vi "ATF Drive and PPSU Feedback.vi"() -> ()   [LabVIEW 2022 SP3]
uses:
  <vilib>/Analysis/baseanly.llb/Mean (DBL).vi
  <vilib>/Analysis/NI_AALBase.lvlib
panel:
  in  "Exit":bool
  out "Deceleration State":bool
  out "Steady State":bool
  out "Accereleration State":bool
  out "C-Phase short circuit":bool
  out "B-Phase short circuit":bool
  out "Motor Winding\n Short circuit or Overload":bool
  out "Speed command &\n response mismatch":bool
  out "C-Phase bottom \nMOSFETshort circuit":bool
  out "C-Phase top\n MOSFET short circuit":bool
  out "B-Phase bottom \nMOSFET short circuit":bool
  out "B-Phase top\n MOSFET short circuit":bool
  out "A-Phase bottom\n MOSFET short  circuit":bool
  out "A-Phase top \nMOSFET short circuit":bool
  out "Over speed":bool
  out "A-Phase short circuit":bool
  out "C-Phase open circuit":bool
  out "B-Phase open circuit":bool
  out "A-Phase open circuit":bool
  out "C-Phase bottom\n MOSFET open circuit":bool
  out "C-Phase top\n MOSFET open circuit":bool
  out "B-Phase bottom \nMOSFET open circuit":bool
  out "B-Phase top \nMOSFET open circuit":bool
  out "A-Phase bottom \nMOSFETopen circuit":bool
  out "A-Phase top\n MOSFET open circuit":bool
  out "Over Temperature":bool
  out "Drive Health":bool
  out "Shaft Rotational Direction":string
  out "Running Frequency":dbl format="%.2f"
  out "Run_Acknowledgement":bool
  out "Speed (RPM)":dbl format="%.2f"
  out "DC Busbar":dbl format="%.2f"
  out "DC Busbar":dbl format="%.2f"
  out "DC Busbar":dbl format="%.2f"
  out "Leg3 Cooling Jacket":dbl format="%.2f"
  out "Leg3 Cooling Jacket":dbl format="%.2f"
  out "Leg2 Cooling Jacket":dbl format="%.2f"
  out "Leg2 Cooling Jacket":dbl format="%.2f"
  out "Leg1 Cooling Jacket":dbl format="%.2f"
  out "Ic,ph,mean":dbl format="%.2f"
  out "Ib,ph,mean":dbl format="%.2f"
  out "Ia,ph,mean":dbl format="%.2f"
  out "Vc,ph,mean":dbl format="%#.2f"
  out "Vb,ph,mean":dbl format="%#.2f"
  out "Va,ph,mean":dbl format="%#.2f"
  out "Ic,ph,rms":dbl format="%.2f"
  out "Ib,ph,rms":dbl format="%.2f"
  out "Ia,ph,rms":dbl format="%.2f"
  out "Idc (A)":dbl format="%.2f"
  out "Vc,ph,rms":dbl format="%.2f"
  out "Vb,ph,rms":dbl format="%.2f"
  out "Va,ph,rms":dbl format="%.2f"
  out "Vdc (V)":dbl format="%.2f"
  # "ATF DRIVE AND PPSU FEEDBACK"
  # "DRIVE HEALTH & FEED BACK"
  # "FAULT STATUS"
  # "Drive Critical Parameters"
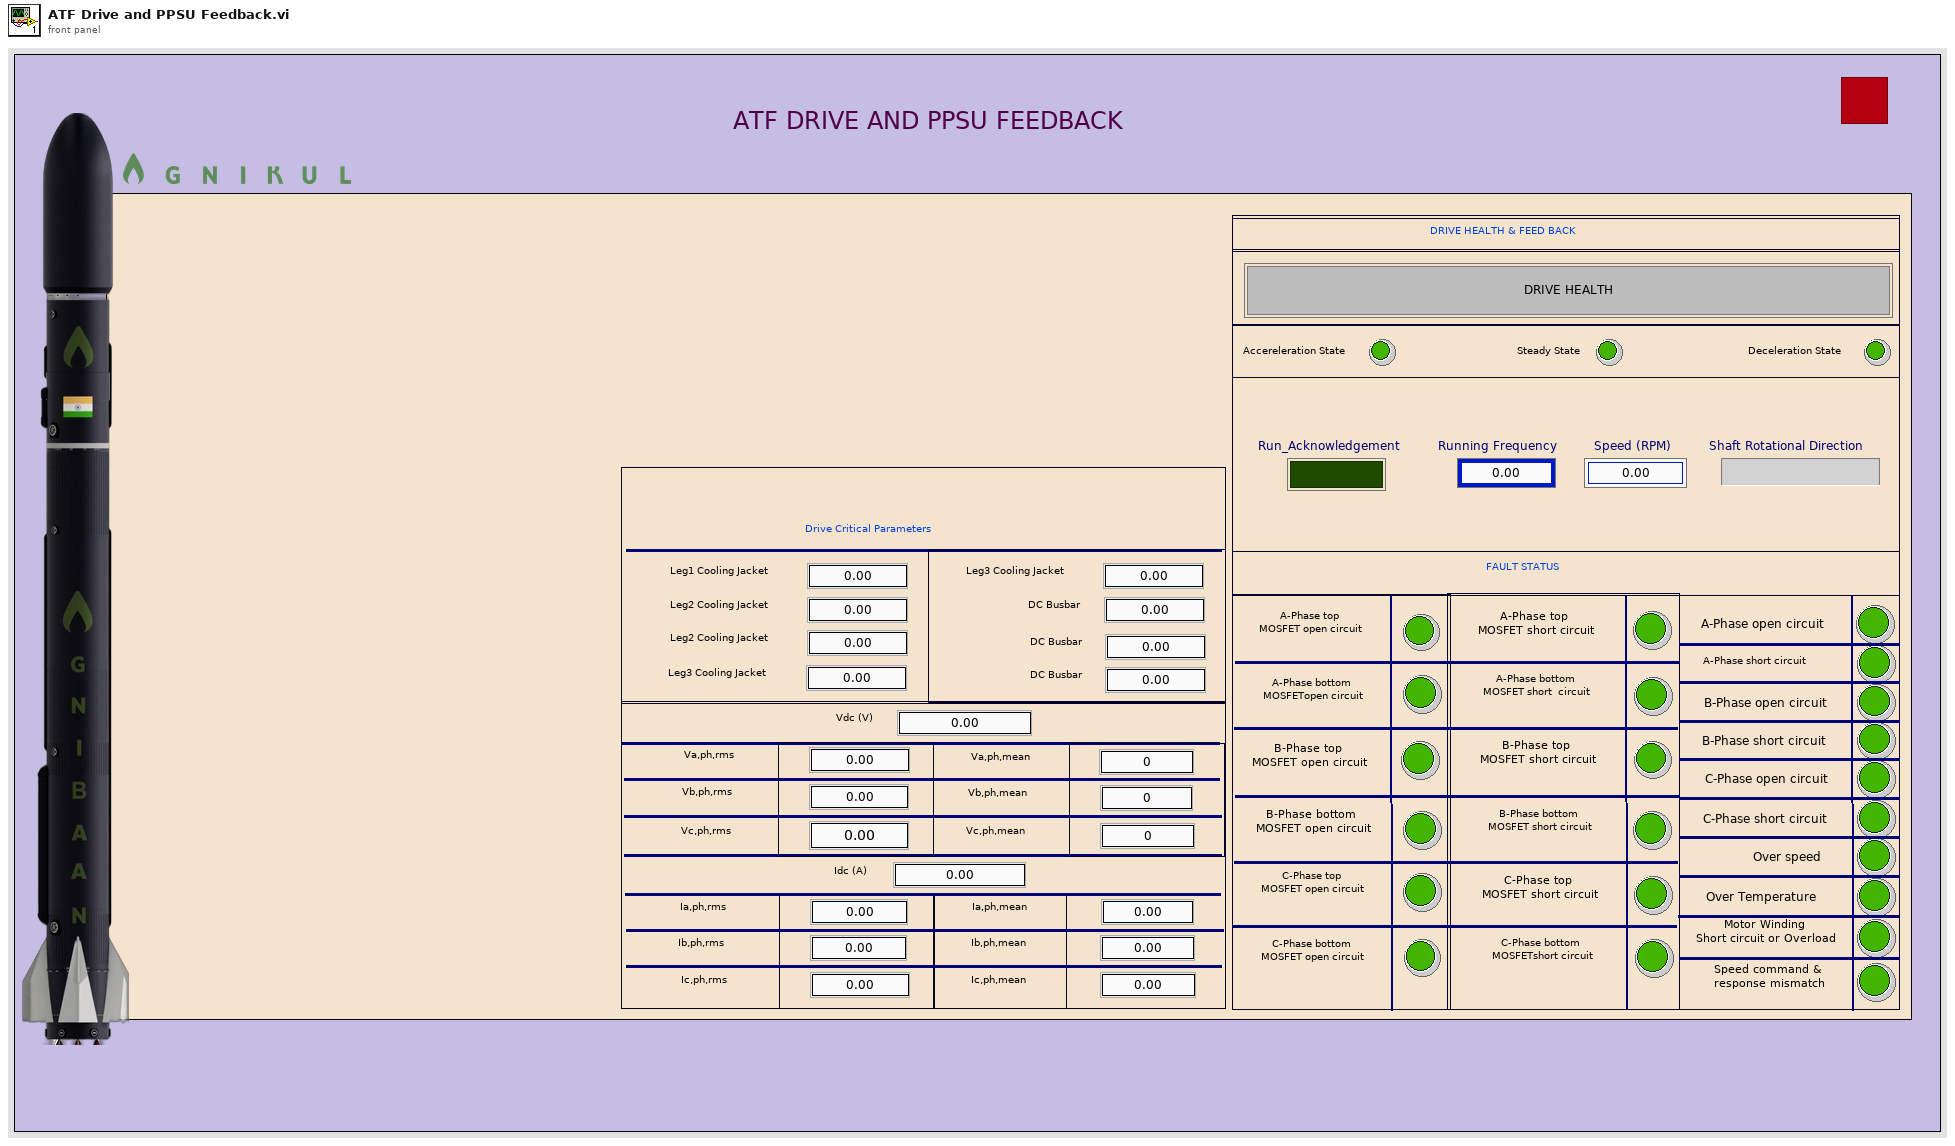
[diagram p1: front panel]
types:
  T1 = typedef "SeCrTS-Notifier Ref.ctl" = cluster{"Pump":refnum<notifier>, "Storage":refnum<notifier>}
  T2 = cluster{"AI_V_Data":waveform(dbl)[][], "AI_C_Data":waveform(dbl)[][], "AO_Data":waveform(dbl)[][], "DO_Data":waveform(dbl)[][], "DI_Data":digitalwaveform[][], "ACC_Data":waveform(dbl)[][], "TC Data":waveform(dbl)[][], "Drive_A_C":waveform(dbl)[][], "Drive_A_D":waveform(dbl)[][], "AI_V Rms":waveform(dbl)[][]}
  T3 = cluster{"Drive_Health":bool, "Drive_Frequency":u32, "Drive_Status":bool, "Drive_RPM":u32, "Drive_Direction":bool, "Acceleration state":bool, "Steady state":bool, "Deceleration state":bool, "Drive_Enable":bool, "Drive set_RPM":dbl}
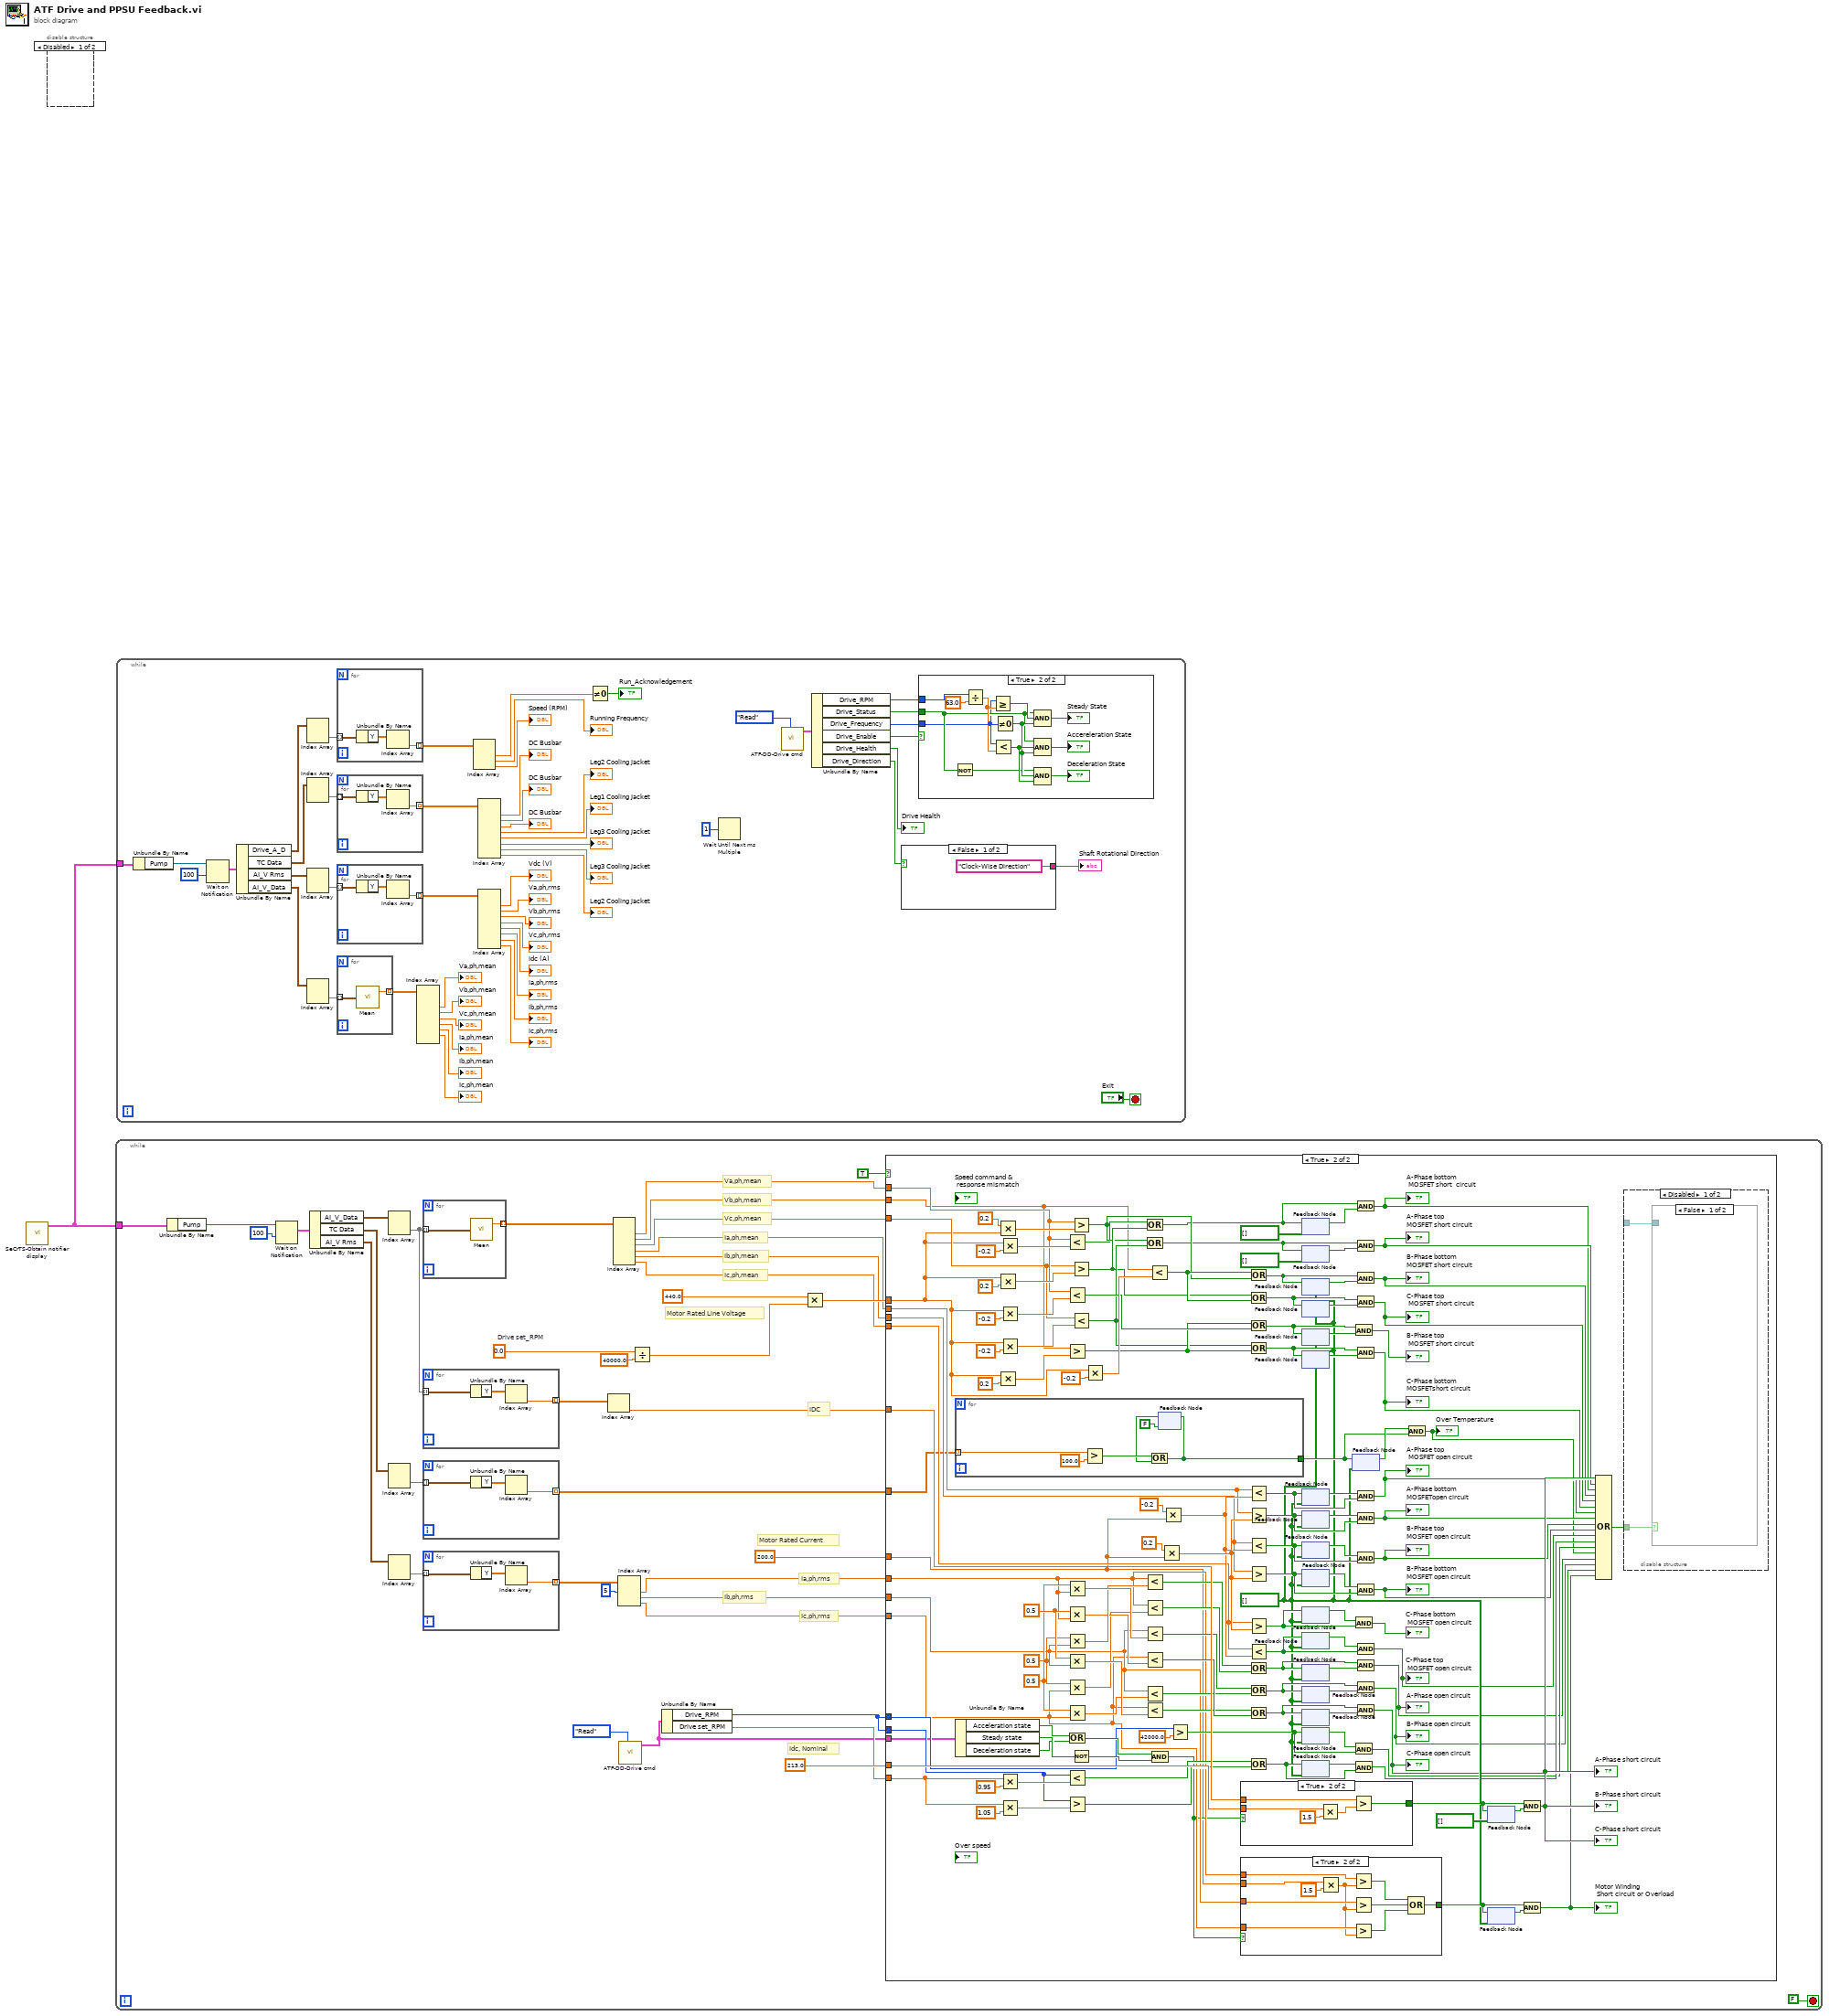
[diagram p0: block diagram]
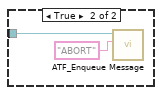
[diagram p3: hidden frame]
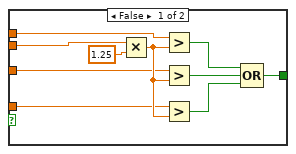
[diagram p5: hidden frame]
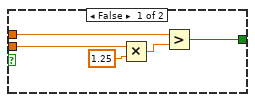
[diagram p6: hidden frame]
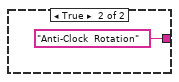
[diagram p9: hidden frame]
diagram:
  n1 = call "SeCrTS-Obtain notifier display.vi"() -> ("NOT DIS Out"=w1:T1)  [unwired: 10 in, 1 out]
  n2 = disable-structure shown="Disabled" {
    frame Disabled {
    }
    frame Enabled {
    }
  }
  n3 = while {
    tunnel: w1 -> [w31]
    stop <- FALSE ("UI Exit") stop-if-true
    w26 = 0.0  # Drive set_RPM
    # "Ic,ph,rms"
    # "Ib,ph,rms"
    # "Ia,ph,rms"
    # "Ic,ph,mean"
    # "Ib,ph,mean"
    # "Ia,ph,mean"
    # "Vb,ph,mean"
    # "Vc,ph,mean"
    # "Va,ph,mean"
    # "IDC"
    # "Idc, Nominal"
    # "Motor Rated Line Voltage"
    # "Motor Rated Current"
    n4 = Unbundle By Name(w31) -> ("Pump"=w30:refnum<notifier>)
    n5 = Wait on Notification(notifier=w30, timeout in ms (-1)=100) -> (notification=w29:T2)  [unwired: 2 in, 3 out]
    n6 = Unbundle By Name(w29) -> ("AI_V_Data"=w28:waveform(dbl)[][], "TC Data"=w25:waveform(dbl)[][], "AI_V Rms"=w13:waveform(dbl)[][])
    n7 = Index Array(array=w28) -> (element=w21:waveform(dbl)[])  [unwired: 2 in]
    n8 = Index Array(array=w25) -> (element=w24:waveform(dbl)[])  [unwired: 2 in]
    n9 = Index Array(array=w13) -> (element=w12:waveform(dbl)[])  [unwired: 2 in]
    n10 = for {
      tunnel: w21 -> [w44] mode=indexing
      tunnel: [w43] -> w20 mode=indexing
      n11 = call-poly <vilib>:"Mean.vi"("X"=w44) -> ("mean"=w43:dbl)  [unwired: 1 out]
    }
    n12 = for {
      tunnel: w21 -> [w47] mode=indexing
      tunnel: [w45] -> w22 mode=indexing
      n13 = Unbundle By Name(w47) -> ("Y"=w46:dbl[])
      n14 = Index Array(array=w46) -> (element=w45:dbl)  [unwired: 1 in]
    }
    n15 = for {
      tunnel: w24 -> [w50] mode=indexing
      tunnel: [w48] -> w35 mode=indexing
      n16 = Unbundle By Name(w50) -> ("Y"=w49:dbl[])
      n17 = Index Array(array=w49) -> (element=w48:dbl)  [unwired: 1 in]
    }
    n18 = for {
      tunnel: w12 -> [w42] mode=indexing
      tunnel: [w40] -> w11 mode=indexing
      n19 = Unbundle By Name(w42) -> ("Y"=w41:dbl[])
      n20 = Index Array(array=w41) -> (element=w40:dbl)  [unwired: 1 in]
    }
    n21 = Index Array(array=w22) -> (element=w27:dbl)  [unwired: 1 in]
    n22 = Index Array(array=w20) -> (element #1=w19:dbl, element #2=w18:dbl, element #3=w17:dbl, element #4=w16:dbl, element #5=w15:dbl, element #6=w14:dbl)  [unwired: 6 in]
    n23 = Index Array(array=w11, index #1=5 ("index")) -> (element #1=w9:dbl, element #2=w8:dbl, element #3=w7:dbl)  [unwired: 2 in]
    n24 = call "ATF-DD-Drive cmd.vi"("Enum"=enum16{"Read", "Write"}."Read") -> ("Data.Drive 2"=w2:T3)  [unwired: 9 in, 1 out]
    n25 = Divide(x=w26, y=40000.0) -> (x/y=w37:dbl)
    n26 = Unbundle By Name(w2) -> ("Drive_RPM"=w6:u32, "Drive set_RPM"=w5:dbl)
    n27 = Multiply(x=440.0, y=w37) -> (x*y=w36:dbl)
    n28 = case shown="True" TRUE {
      tunnel: 213.0 -> [_ w181]
      tunnel: w27 -> [_ w180]
      tunnel: w19 -> [_ w158]
      tunnel: w17 -> [_ w157]
      tunnel: w18 -> [_ w156]
      tunnel: w36 -> [_ w155]
      tunnel: w16 -> [_ w135]
      tunnel: w15 -> [_ w134]
      tunnel: w14 -> [_ w133]
      tunnel: w6 -> [_ w113]
      tunnel: w6 -> [_ w109]
      tunnel: w35 -> [_ w106]
      tunnel: w9 -> [_ w82]
      tunnel: w8 -> [_ w81]
      tunnel: w7 -> [_ w80]
      tunnel: 200.0 -> [_ w75]
      tunnel: w2 -> [_ w55]
      tunnel: w5 -> [_ w51]
      frame False {
      }
      frame True {
        w97 = 0.5 ("upper limit")
        w96 = 0.5 ("upper limit")
        w89 = 0.5 ("upper limit")
        w76 = bool[] []
        n29 = for {
          tunnel: [w211] -> w104
          tunnel: w106 -> [w212] mode=indexing
          n30 = Greater?(x=w212, y=100.0) -> (0:w215:bool)
          n31 = feedback #1(FALSE) -> (w214:bool)
          n32 = Or(x=w215, y=w214) -> (x .or. y?=w211:bool)
          n33 = feedback-in #1(w211) -> ()
        }
        n34 = Unbundle By Name(w55) -> ("Acceleration state"=w54:bool, "Steady state"=w53:bool, "Deceleration state"=w52:bool)
        n35 = Multiply(x=0.2 ("y"), y=w155) -> (x*y=w169:dbl)
        n36 = Multiply(x=w155, y=0.2) -> (x*y=w172:dbl)
        n37 = Multiply(x=w155, y=0.2) -> (x*y=w173:dbl)
        n38 = Multiply(x=w155, y=-0.2) -> (x*y=w170:dbl)
        n39 = Multiply(x=w155, y=-0.2) -> (x*y=w175:dbl)
        n40 = Multiply(x=w155, y=-0.2) -> (x*y=w171:dbl)
        n41 = Multiply(x=w51, y=0.95) -> (x*y=w117:dbl)
        n42 = Multiply(x=w51, y=1.05) -> (x*y=w116:dbl)
        n43 = Less?(x=w158, y=w170) -> (x < y?=w163:bool)
        n44 = Less?(x=w158, y=w175) -> (x < y?=w176:bool)
        n45 = Greater?(x=w156, y=w173) -> (0:w168:bool)
        n46 = Multiply(x=w96, y=w82) -> (x*y=w102:dbl)
        n47 = Multiply(x=w97, y=w82) -> (x*y=w98:dbl)
        n48 = Multiply(x=w89, y=w81) -> (x*y=w101:dbl)
        n49 = Multiply(x=w97, y=w81) -> (x*y=w103:dbl)
        n50 = Multiply(x=w89, y=w80) -> (x*y=w90:dbl)
        n51 = Multiply(x=w96, y=w80) -> (x*y=w95:dbl)
        n52 = Or(x=w54, y=w52) -> (x .or. y?=w183:bool)
        n53 = Less?(x=w113, y=w117) -> (x < y?=w118:bool)
        n54 = Greater?(x=w113, y=w116) -> (0:w119:bool)
        n55 = Greater?(x=w158, y=w169) -> (0:w165:bool)
        n56 = Greater?(x=w157, y=w172) -> (0:w166:bool)
        n57 = Less?(x=w157, y=w171) -> (x < y?=w167:bool)
        n58 = Not(x=w53) -> (.not. x?=w182:bool)
        n59 = Multiply(x=w155, y=-0.2) -> (x*y=w177:dbl)
        n60 = Or(x=w163, y=w166) -> (x .or. y?=w145:bool)
        n61 = Or(x=w165, y=w167) -> (x .or. y?=w146:bool)
        n62 = Less?(x=w82, y=w101) -> (x < y?=w91:bool)
        n63 = Less?(x=w82, y=w90) -> (x < y?=w92:bool)
        n64 = Less?(x=w81, y=w102) -> (x < y?=w94:bool)
        n65 = Less?(x=w80, y=w98) -> (x < y?=w100:bool)
        n66 = Less?(x=w81, y=w95) -> (x < y?=w93:bool)
        n67 = Less?(x=w80, y=w103) -> (x < y?=w99:bool)
        n68 = Less?(x=w156, y=w177) -> (x < y?=w179:bool)
        n69 = And(x=w183, y=w182) -> (x .and. y?=w79:bool)
        n70 = Multiply(x=0.2 ("y"), y=w75) -> (x*y=w139:dbl)
        n71 = Multiply(x=-0.2 ("y"), y=w75) -> (x*y=w137:dbl)
        n72 = Greater?(x=w109, y=42000.0) -> (0:w107:bool)
        n73 = case shown="True" w79 {
          tunnel: [w220 w225] -> w186
          tunnel: w181 -> [w218 w223]
          tunnel: w180 -> [w217 w222]
          frame False {
            n74 = Multiply(x=w218, y=1.25) -> (x*y=w219:dbl)
            n75 = Greater?(x=w217, y=w219) -> (0:w220:bool)
          }
          frame True {
            n76 = Multiply(x=w223, y=1.5) -> (x*y=w224:dbl)
            n77 = Greater?(x=w222, y=w224) -> (0:w225:bool)
          }
        }
        n78 = case shown="True" w79 {
          tunnel: w82 -> [w192 w210]
          tunnel: w81 -> [w194 w209]
          tunnel: w80 -> [w195 w208]
          tunnel: [w191 w204] -> w77
          tunnel: w75 -> [w193 w203]
          frame False {
            n79 = Multiply(x=w193, y=1.25) -> (x*y=w196:dbl)
            n80 = Greater?(x=w192, y=w196) -> (0:w200:bool)
            n81 = Greater?(x=w194, y=w196) -> (0:w199:bool)
            n82 = Greater?(x=w195, y=w196) -> (0:w198:bool)
            n83 = Compound Arithmetic op=OR(w200, w199, w198) -> (w191:bool)
          }
          frame True {
            n84 = Multiply(x=w203, y=1.5) -> (x*y=w201:dbl)
            n85 = Greater?(x=w210, y=w201) -> (0:w207:bool)
            n86 = Greater?(x=w209, y=w201) -> (0:w206:bool)
            n87 = Greater?(x=w208, y=w201) -> (0:w205:bool)
            n88 = Compound Arithmetic op=OR(w207, w206, w205) -> (w204:bool)
          }
        }
        n89 = Or(x=w179, y=w165) -> (x .or. y?=w143:bool)
        n90 = Or(x=w166, y=w179) -> (x .or. y?=w142:bool)
        n91 = Or(x=w168, y=w176) -> (x .or. y?=w144:bool)
        n92 = Or(x=w167, y=w168) -> (x .or. y?=w141:bool)
        n93 = Less?(x=w135, y=w137) -> (x < y?=w121:bool)
        n94 = Greater?(x=w135, y=w139) -> (0:w122:bool)
        n95 = Less?(x=w134, y=w137) -> (x < y?=w123:bool)
        n96 = Greater?(x=w134, y=w139) -> (0:w124:bool)
        n97 = Greater?(x=w133, y=w139) -> (0:w126:bool)
        n98 = Less?(x=w133, y=w137) -> (x < y?=w125:bool)
        n99 = Or(x=w91, y=w92) -> (x .or. y?=w83:bool)
        n100 = Or(x=w94, y=w93) -> (x .or. y?=w84:bool)
        n101 = Or(x=w99, y=w100) -> (x .or. y?=w85:bool)
        n102 = Or(x=w118, y=w119) -> (x .or. y?=w111:bool)
        n103 = feedback #2(bool[] []) -> (w150:bool)
        n104 = feedback-in #2(w145) -> ()
        n105 = feedback #3(bool[] []) -> (w148:bool)
        n106 = feedback-in #3(w146) -> ()
        n107 = feedback #4(w76) -> (w152:bool)
        n108 = feedback-in #4(w143) -> ()
        n109 = feedback #5(w76) -> (w153:bool)
        n110 = feedback-in #5(w142) -> ()
        n111 = feedback #6(w76) -> (w151:bool)
        n112 = feedback-in #6(w144) -> ()
        n113 = feedback #7(w76) -> (w154:bool)
        n114 = feedback-in #7(w141) -> ()
        n115 = feedback #8(w76) -> (w131:bool)
        n116 = feedback-in #8(w121) -> ()
        n117 = feedback #9(w76) -> (w130:bool)
        n118 = feedback-in #9(w122) -> ()
        n119 = feedback #10(w76) -> (w129:bool)
        n120 = feedback-in #10(w123) -> ()
        n121 = feedback #11(w76) -> (w128:bool)
        n122 = feedback-in #11(w124) -> ()
        n123 = feedback #12(w76) -> (w132:bool)
        n124 = feedback-in #12(w126) -> ()
        n125 = feedback #13(w76) -> (w127:bool)
        n126 = feedback-in #13(w125) -> ()
        n127 = feedback #14(w76) -> (w86:bool)
        n128 = feedback-in #14(w83) -> ()
        n129 = feedback #15(w76) -> (w87:bool)
        n130 = feedback-in #15(w84) -> ()
        n131 = feedback #16(w76) -> (w88:bool)
        n132 = feedback-in #16(w85) -> ()
        n133 = feedback #17(w76) -> (w108:bool)
        n134 = feedback-in #17(w107) -> ()
        n135 = feedback #18(w76) -> (w112:bool)
        n136 = feedback-in #18(w111) -> ()
        n137 = feedback #19(w76) -> (w105:bool)
        n138 = feedback-in #19(w104) -> ()
        n139 = And(x=w144, y=w151) -> (x .and. y?=→"B-Phase top\n MOSFET short circuit":bool)
        n140 = And(x=w132, y=w126) -> (x .and. y?=→"C-Phase bottom\n MOSFET open circuit":bool)
        n141 = And(x=w108, y=w107) -> (x .and. y?=w62:bool)
        n142 = And(x=w112, y=w111) -> (x .and. y?=w63:bool)
        n143 = And(x=w145, y=w150) -> (x .and. y?=w72:bool)
        "A-Phase bottom\n MOSFET short  circuit" <- w72
        n144 = And(x=w146, y=w148) -> (x .and. y?=w73:bool)
        "A-Phase top \nMOSFET short circuit" <- w73
        n145 = And(x=w143, y=w152) -> (x .and. y?=w71:bool)
        "B-Phase bottom \nMOSFET short circuit" <- w71
        n146 = And(x=w142, y=w153) -> (x .and. y?=w70:bool)
        "C-Phase top\n MOSFET short circuit" <- w70
        n147 = And(x=w141, y=w154) -> (x .and. y?=w69:bool)
        "C-Phase bottom \nMOSFETshort circuit" <- w69
        n148 = And(x=w131, y=w121) -> (x .and. y?=w68:bool)
        "A-Phase top\n MOSFET open circuit" <- w68
        n149 = And(x=w130, y=w122) -> (x .and. y?=w67:bool)
        "A-Phase bottom \nMOSFETopen circuit" <- w67
        n150 = And(x=w129, y=w123) -> (x .and. y?=w66:bool)
        "B-Phase top \nMOSFET open circuit" <- w66
        n151 = And(x=w128, y=w124) -> (x .and. y?=w65:bool)
        "B-Phase bottom \nMOSFET open circuit" <- w65
        n152 = And(x=w127, y=w125) -> (x .and. y?=w64:bool)
        "C-Phase top\n MOSFET open circuit" <- w64
        n153 = And(x=w83, y=w86) -> (x .and. y?=w60:bool)
        "A-Phase open circuit" <- w60
        n154 = And(x=w84, y=w87) -> (x .and. y?=w59:bool)
        "B-Phase open circuit" <- w59
        n155 = And(x=w85, y=w88) -> (x .and. y?=w58:bool)
        "C-Phase open circuit" <- w58
        n156 = And(x=w105, y=w104) -> (x .and. y?=w61:bool)
        "Over Temperature" <- w61
        n157 = feedback #20(bool[] []) -> (w185:bool)
        n158 = feedback-in #20(w186) -> ()
        n159 = feedback #21(w76) -> (w78:bool)
        n160 = feedback-in #21(w77) -> ()
        n161 = And(x=w186, y=w185) -> (x .and. y?=w74:bool)
        "A-Phase short circuit" <- w74
        "B-Phase short circuit" <- w74
        "C-Phase short circuit" <- w74
        n162 = And(x=w77, y=w78) -> (x .and. y?=w57:bool)
        "Motor Winding\n Short circuit or Overload" <- w57
        n163 = Compound Arithmetic op=OR(w74, w73, w72, w71, w70, w69, w68, w67, w66, w65, w64, w63, w62, w61, w60, w59, w58, w57) -> (w56:bool)
        n164 = disable-structure shown="Disabled" {
          disable-tunnel: _ -> [w188 _]
          disable-tunnel: w56 -> [w187 _]
          frame Disabled {
            n165 = case shown="False" w187 {
              tunnel: w188 -> [_ w190]
              frame False {
              }
              frame True {
                n166 = call "ATF_Enqueue Message.vi"("Message"="ABORT", "Message Queue"=w190) -> ()  [unwired: 8 in, 2 out]
              }
            }
          }
          frame Enabled {
          }
        }
      }
    }
  }
  n167 = while {
    tunnel: w1 -> [w251]
    stop <- "Exit" stop-if-true
    n168 = Unbundle By Name(w251) -> ("Pump"=w253:refnum<notifier>)
    n169 = Wait on Notification(notifier=w253, timeout in ms (-1)=100) -> (notification=w252:T2)  [unwired: 2 in, 3 out]
    n170 = Unbundle By Name(w252) -> ("Drive_A_D"=w241:waveform(dbl)[][], "TC Data"=w246:waveform(dbl)[][], "AI_V Rms"=w248:waveform(dbl)[][], "AI_V_Data"=w250:waveform(dbl)[][])
    n171 = Index Array(array=w241) -> (element=w240:waveform(dbl)[])  [unwired: 2 in]
    n172 = Index Array(array=w246) -> (element=w245:waveform(dbl)[])  [unwired: 2 in]
    n173 = Index Array(array=w248) -> (element=w247:waveform(dbl)[])  [unwired: 2 in]
    n174 = Index Array(array=w250) -> (element=w249:waveform(dbl)[])  [unwired: 2 in]
    n175 = for {
      tunnel: w240 -> [w294] mode=indexing
      tunnel: [w292] -> w239 mode=indexing
      n176 = Unbundle By Name(w294) -> ("Y"=w293:dbl[])
      n177 = Index Array(array=w293) -> (element=w292:dbl)  [unwired: 1 in]
    }
    n178 = for {
      tunnel: w245 -> [w300] mode=indexing
      tunnel: [w298] -> w268 mode=indexing
      n179 = Unbundle By Name(w300) -> ("Y"=w299:dbl[])
      n180 = Index Array(array=w299) -> (element=w298:dbl)  [unwired: 1 in]
    }
    n181 = for {
      tunnel: [w295] -> w274 mode=indexing
      tunnel: w247 -> [w296] mode=indexing
      n182 = Unbundle By Name(w296) -> ("Y"=w297:dbl[])
      n183 = Index Array(array=w297) -> (element=w295:dbl)  [unwired: 1 in]
    }
    n184 = for {
      tunnel: w249 -> [w302] mode=indexing
      tunnel: [w301] -> w273 mode=indexing
      n185 = call-poly <vilib>:"Mean.vi"("X"=w302) -> ("mean"=w301:dbl)  [unwired: 1 out]
    }
    n186 = Index Array(array=w273) -> (element #2=→"Va,ph,mean":dbl, element #3=→"Vb,ph,mean":dbl, element #4=→"Vc,ph,mean":dbl, element #5=→"Ia,ph,mean":dbl, element #6=→"Ib,ph,mean":dbl, element #7=→"Ic,ph,mean":dbl)  [unwired: 8 in, 2 out]
    n187 = Index Array(array=w239) -> (element #1=w238:dbl, element #2=→"Running Frequency":dbl, element #3=→"Speed (RPM)":dbl)  [unwired: 3 in]
    n188 = Index Array(array=w268) -> (element #1=→"DC Busbar":dbl, element #2=→"DC Busbar":dbl, element #3=→"DC Busbar":dbl, element #4=→"Leg2 Cooling Jacket":dbl, element #5=→"Leg1 Cooling Jacket":dbl, element #6=→"Leg3 Cooling Jacket":dbl, element #7=→"Leg3 Cooling Jacket":dbl, element #8=→"Leg2 Cooling Jacket":dbl)  [unwired: 8 in]
    n189 = Index Array(array=w274) -> (element #1=→"Vdc (V)":dbl, element #2=→"Va,ph,rms":dbl, element #3=→"Vb,ph,rms":dbl, element #4=→"Vc,ph,rms":dbl, element #5=→"Idc (A)":dbl, element #6=→"Ia,ph,rms":dbl, element #7=→"Ib,ph,rms":dbl, element #8=→"Ic,ph,rms":dbl)  [unwired: 8 in]
    n190 = Not Equal To 0?(x=w238) -> (x != 0?=→"Run_Acknowledgement":bool)
    n191 = Wait Until Next ms Multiple(millisecond multiple=u32 1) -> ()  [unwired: 1 out]
    n192 = call "ATF-DD-Drive cmd.vi"("Enum"=enum16{"Read", "Write"}."Read") -> ("Data.Drive 2"=w233:T3)  [unwired: 9 in, 1 out]
    n193 = Unbundle By Name(w233) -> ("Drive_RPM"=w230:u32, "Drive_Status"=w229:bool, "Drive_Frequency"=w228:u32, "Drive_Enable"=w231:bool, "Drive_Health"=→"Drive Health":bool, "Drive_Direction"=w227:bool)
    n194 = case shown="False" w227 {
      tunnel: ["Clock-Wise Direction" ("Shaft Rotational Direction") "Anti-Clock  Rotation" ("Shaft Rotational Direction")] -> w244
      frame False {
      }
      frame True {
      }
    }
    "Shaft Rotational Direction" <- w244
    n195 = case shown="True" w231 {
      tunnel: w230 -> [_ w285]
      tunnel: w229 -> [_ w284]
      tunnel: w228 -> [_ w283]
      frame False {
      }
      frame True {
        n196 = Not(x=w284) -> (.not. x?=w288:bool)
        n197 = Divide(x=w285, y=63.0 ("x")) -> (x/y=w286:dbl)
        n198 = Greater Or Equal?(x=w283, y=w286) -> (x >= y?=w291:bool)
        n199 = Less?(x=w283, y=w286) -> (x < y?=w290:bool)
        n200 = Not Equal To 0?(x=w283) -> (x != 0?=w289:bool)
        n201 = Compound Arithmetic op=AND(w284, w291, w289) -> (→"Steady State":bool)
        n202 = Compound Arithmetic op=AND(w284, w290, w289) -> (→"Accereleration State":bool)
        n203 = Compound Arithmetic op=AND(w288, w289, w290) -> (→"Deceleration State":bool)
      }
    }
  }
